vi "ATE_BSE-Event_Dequeue.vi"(8 "error in (no error)":errorcluster) -> (0 "error out":errorcluster, 3 "Event":T1)   [LabVIEW 2021]
uses:
  Controls/ATE_BSE_Event_type_def.ctl
  Controls/ATE_BSE_Queue_Operations.ctl
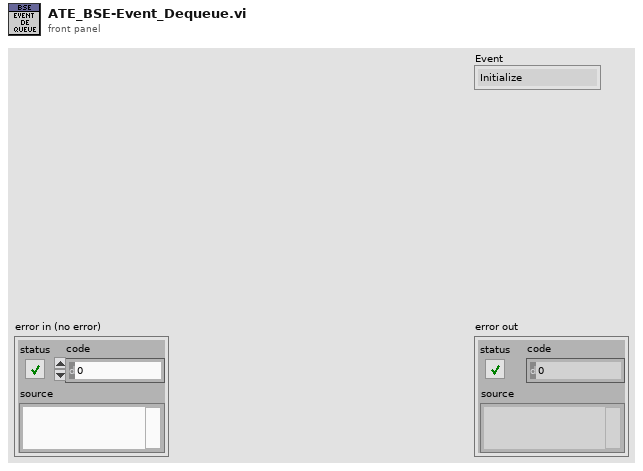
[diagram p1: front panel]
types:
  T1 = typedef "ATE_BSE_Event_type_def.ctl" = enum16{"Initialize", "Configure", "Ip Simulation", "UE-Display", "IMS", "Sim Configurations", "ECall", "Exit", "Error"}
  T2 = typedef "ATE_BSE_Queue_Operations.ctl" = enum16{"Init", "Get Queue", "Flush", "Close"}
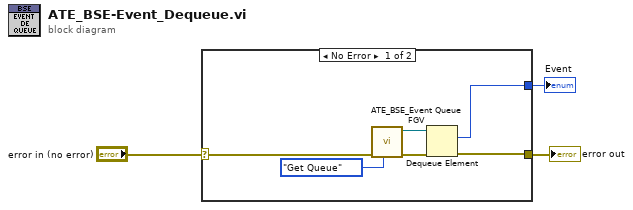
[diagram p0: block diagram]
diagram:
  n1 = case shown="No Error" "error in (no error)" {
    selector: "error in (no error)" -> [w9 w10]
    tunnel: [w6 w10] -> w3
    tunnel: [w5 _] -> w1
    frame No Error {
      n2 = call "ATE_BSE_Event Queue FGV.vi"("Operations"=ATE_BSE_Queue_Operations."Get Queue", "error in (no error)"=w9) -> ("error out"=w8:errorcluster, "queue out"=w7:refnum<queue>)  [unwired: 8 in]
      n3 = Dequeue Element(queue=w7, error in (no error)=w8) -> (element=w5:T1, error out=w6:errorcluster)  [unwired: 1 in, 2 out]
    }
    frame Error {
    }
  }
  "error out" <- w3
  "Event" <- w1
